vi "linearAccumulator.vi"(6 "reset":bool, 7 "inputValid":bool, 10 "input":i16) -> (0 "outputValid":bool, 3 "sum":i32)   [LabVIEW 2016]
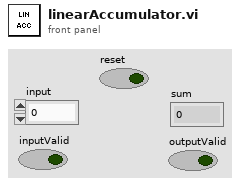
[diagram p1: front panel]
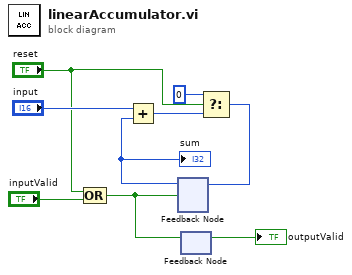
[diagram p0: block diagram]
diagram:
  n1 = Compound Arithmetic op=OR("reset", "inputValid") -> (w3:bool)
  n2 = feedback #1() -> (w1:i32)  [unwired: 1 in]
  "sum" <- w1
  n3 = Add(x="input", y=w1) -> (x+y=w9:i32)
  n4 = feedback-in #2(w3) -> ()
  n5 = feedback #2() -> (→"outputValid":bool)  [unwired: 1 in]
  n6 = Select(t=0, s="reset", f=w9) -> (s? t:f=w7:i32)
  n7 = feedback-in #1(w7, w3) -> ()
